vi "calcDemandedSteps.vi"(8 "error in (no error)":errorcluster, 11 "Model in":refnum<class "Model.lvclass">) -> (0 "error out":errorcluster, 3 "Model out":refnum<class "Model.lvclass">)   [LabVIEW 2013, in "Model.lvclass"]
uses:
  Model.lvclass
  ApplicationElements/SystemController/SystemController.lvclass
  <userlib>/Common/ILC/ILC/ILC.lvclass
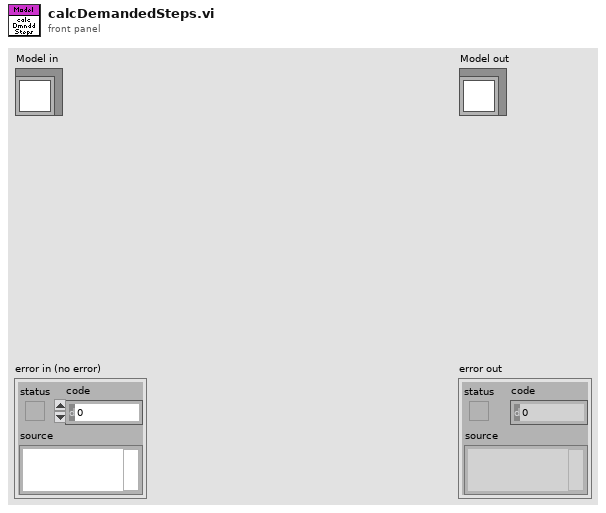
[diagram p1: front panel]
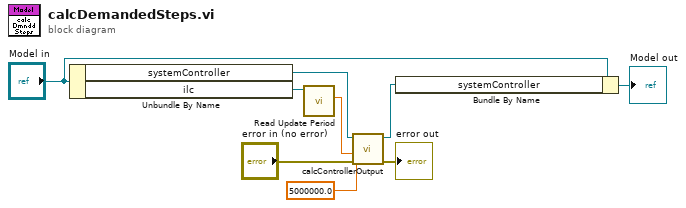
[diagram p0: block diagram]
diagram:
  n1 = Unbundle By Name("Model in") -> ("systemController"=w5:refnum<class "SystemController.lvclass">, "ilc"=w3:refnum<class "ILC.lvclass">)
  n2 = call <userlib>:"Read Update Period.vi"("ILC in"=w3) -> ("Update Period"=w2:dbl[unit])  [unwired: 9 in, 1 out]
  n3 = call "calcControllerOutput.vi"("error in (no error)"="error in (no error)", "loopPeriod"=w2, "step rate limit (mag)"=dbl[unit] 5000000.0, "SystemController in"=w5) -> ("error out"=→"error out":errorcluster, "SystemController out"=w4:refnum<class "SystemController.lvclass">)  [unwired: 5 in, 1 out]
  n4 = Bundle By Name(cluster="Model in", "systemController"=w4) -> (→"Model out":refnum<class "Model.lvclass">)
